vi "STM Get Connection Reference (Serial).vi"(8 "error in":errorcluster, 11 "Connection Info":T1) -> (0 "error out":errorcluster, 2 "VISA resource name out":refnum<visa-resource-name>, 3 "Connection Info Out":T1)   [LabVIEW 2010]
doc: "Returns the serial VISA reference."
uses:
  stm_Serial Connection Info.ctl
  stm_MetaDataElement.ctl
  NI STM.lvlib
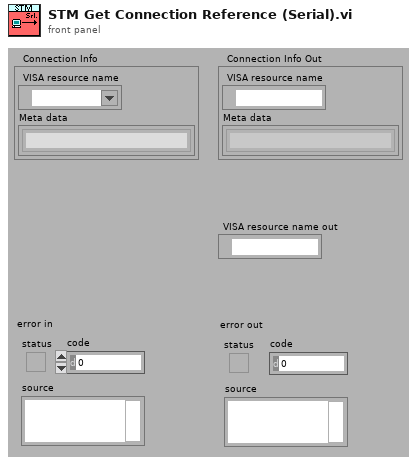
[diagram p1: front panel]
types:
  T1 = typedef "stm_Serial Connection Info.ctl" = cluster{"VISA resource name":refnum<visa-resource-name>, "Meta data":T2[]}
  T2 = typedef "stm_MetaDataElement.ctl" = string
  T3 = typedef "NI STM.lvlib/Serial Connection Info.ctl" = cluster{"VISA resource name":refnum<visa-resource-name>, "Meta data":T4[]}
  T4 = typedef "NI STM.lvlib/MetaDataElement.ctl" = string
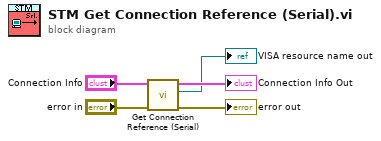
[diagram p0: block diagram]
diagram:
  n1 = call "Get Connection Reference (Serial).vi"("error in"="error in", "Connection Info In"="Connection Info") -> ("error out"=→"error out":errorcluster, "VISA resource name out"=→"VISA resource name out":refnum<visa-resource-name>, "Connection Info Out"=→"Connection Info Out":T3)  [unwired: 7 in]
